vi "GetEquipmentProperties.vi"(9 "Device":bool, 10 "EquipmentIds":string[](array[string]), 11 "Equipment List":T2[](array[typedef])) -> (2 "Tdms Properties":T1[](array[typedef]))   [LabVIEW 2017, in "Tdms.lvlib"]
uses:
  <vilib>/addons/InsightCM/Utilities/Tdms/Tdms.lvlib
  <vilib>/addons/InsightCM/MessageBus/Base/controls/Equipment.ctl
  <vilib>/addons/InsightCM/MessageBus/Base/controls/KeyValuePair.ctl
  <vilib>/addons/InsightCM/Utilities/Tdms/controls/Property.ctl
  <vilib>/addons/InsightCM/Utilities/DeviceModelHelpers/DeviceModelHelpers.lvlib
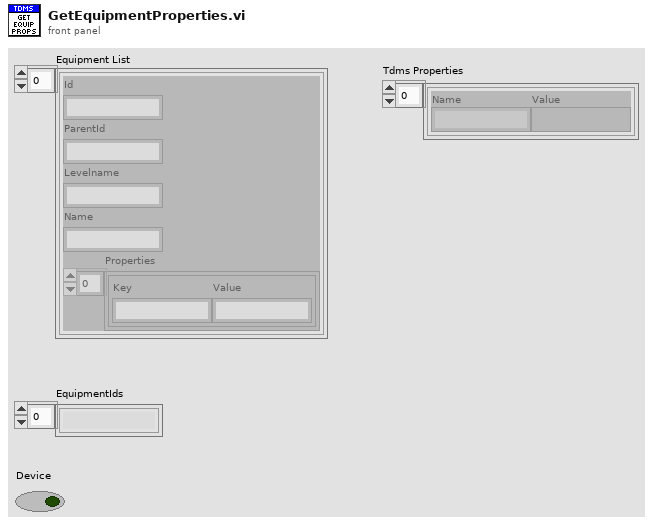
[diagram p1: front panel]
types:
  T1 = typedef "Tdms.lvlib/Property.ctl" = cluster{"Name":string, "Value":variant}
  T2 = typedef "Equipment.ctl" = cluster{"Id":string, "ParentId":string, "Levelname":string, "Name":string, "Properties":T3[]}
  T3 = typedef "KeyValuePair.ctl" = cluster{"Key":string, "Value":string}
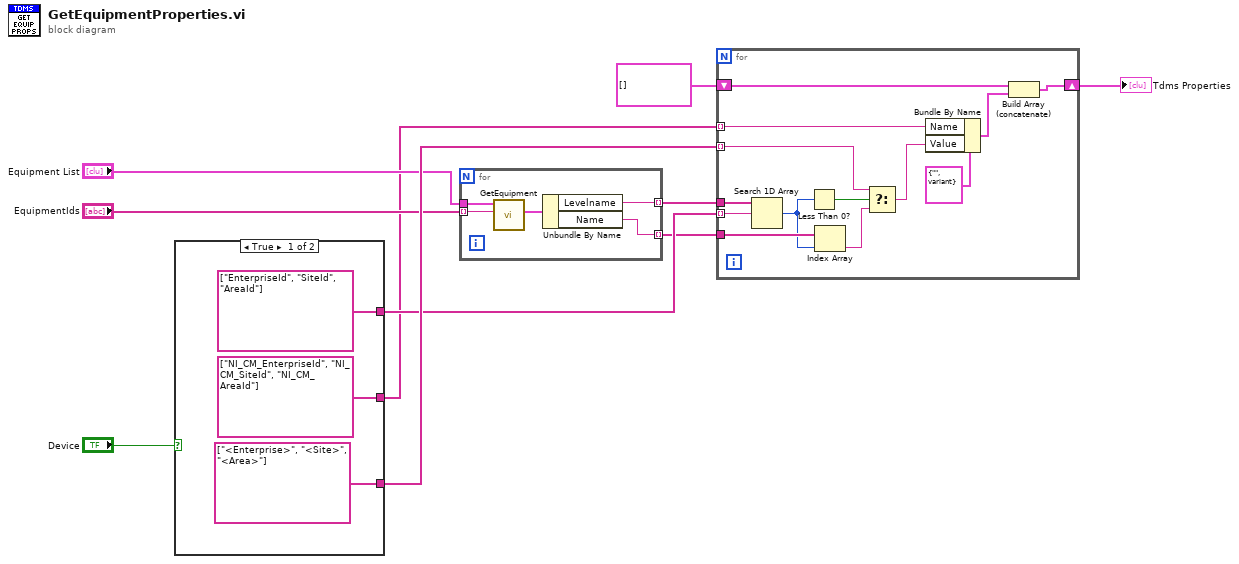
[diagram p0: block diagram]
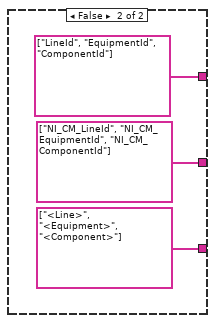
[diagram p2: hidden frame]
diagram:
  n1 = case shown="True" "Device" {
    tunnel: [string[] ["EnterpriseId", "SiteId", "AreaId"] string[] ["LineId", "EquipmentId", "ComponentId"]] -> w5
    tunnel: [string[] ["NI_CM_EnterpriseId", "NI_CM_SiteId", "NI_CM_AreaId"] string[] ["NI_CM_LineId", "NI_CM_EquipmentId", "NI_CM_ComponentId"]] -> w3
    tunnel: [string[] ["<Enterprise>", "<Site>", "<Area>"] string[] ["<Line>", "<Equipment>", "<Component>"]] -> w9
    frame True {
    }
    frame False {
    }
  }
  n2 = for {
    tunnel: "Equipment List" -> [w21]
    tunnel: "EquipmentIds" -> [w20] mode=indexing
    tunnel: [w18] -> w6 mode=indexing
    tunnel: [w17] -> w4 mode=indexing
    n3 = call <vilib>:"GetEquipment.vi"("id"=w20, "equipment list"=w21) -> ("equipment"=w19:T2)  [unwired: 7 in, 2 out]
    n4 = Unbundle By Name(w19) -> ("Levelname"=w18:string, "Name"=w17:string)
  }
  n5 = for {
    shift-right: [w31] -> w1
    shift-left: T1[] [] -> [w33]
    tunnel: w6 -> [w34]
    tunnel: w4 -> [w32]
    tunnel: w9 -> [w24] mode=indexing
    tunnel: w5 -> [w29] mode=indexing
    tunnel: w3 -> [w27] mode=indexing
    n6 = Search 1D Array(1D array=w34, element=w29) -> (index of element=w28:i32)  [unwired: 1 in]
    n7 = Less Than 0?(x=w28) -> (x < 0?=w26:bool)
    n8 = Index Array(array=w32, index=w28) -> (element=w25:string)
    n9 = Select(t=w24, s=w26, f=w25) -> (s? t:f=w23:string)
    n10 = Bundle By Name(cluster=T1 {"Name"="", "Value"=variant} ("Property"), "Name"=w27, "Value"=w23) -> (w30:T1)
    n11 = Build Array (concatenate)(w33, w30) -> (w31:T1[])
  }
  "Tdms Properties" <- w1
